vi "读取高速数据.vi"(6 "超时毫秒":i32=1000, 8 "错误输入":errorcluster caption="错误输入（无错误）", 10 "数据个数":i32, 11 "设备句柄入":i32) -> (0 "错误输出":errorcluster, 1 "返回数据个数":i32, 2 "原码值":u16[](array[numeric]), 3 "设备句柄":i32=1)   [LabVIEW 2011]
uses:
  dll/em9636.dll
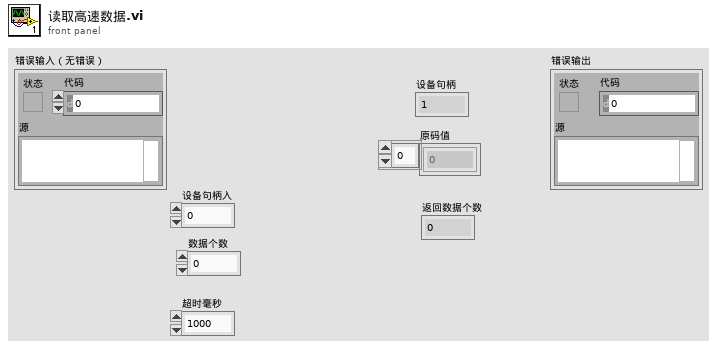
[diagram p1: front panel]
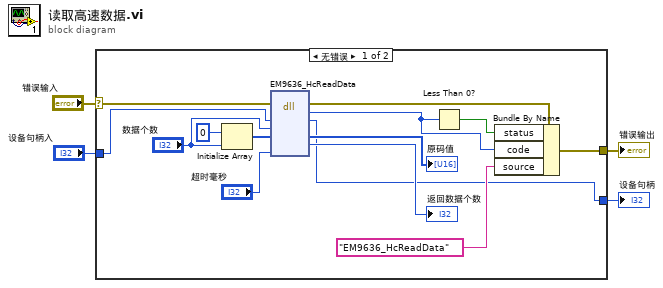
[diagram p0: block diagram]
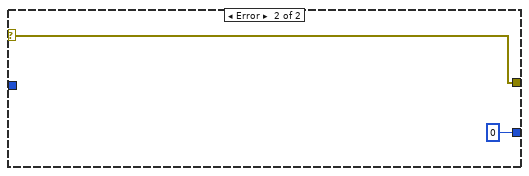
[diagram p2: hidden frame]
diagram:
  n1 = case shown="无错误" "错误输入" {
    selector: "错误输入" -> [w18 w20]
    tunnel: [w14 w20] -> w3
    tunnel: [w5 0 ("错误")] -> w2
    tunnel: "设备句柄入" -> [w12 _]
    frame No Error {
      n2 = Initialize Array(u16 0 ("元素"), "数据个数") -> (w7:u16[])
      n3 = dll-call lib="PTH1abs Eèµ éç LABVIEWæºVI(v2.0)EM9636BD)EM9636BDè°ç¨APIå½æ°æ¹æ³éè®¯ä¾ç¨EM9636labview8.5-1511048.5dll\nem9636.dll" fn="EM9636_HcReadData"(error in=w18, "设备句柄"=w12, "数据个数"="数据个数", "原码值"=w7, "超时毫秒"="超时毫秒") -> (error out=w16:errorcluster, "错误"=w13:i32, "设备句柄"=w5:i32, "原码值"=→"原码值":u16[], "返回数据个数"=→"返回数据个数":i32)  [unwired: 5 in, 1 out]
      n4 = Less Than 0?(x=w13) -> (x < 0?=w15:bool)
      n5 = Bundle By Name(cluster=w16, "status"=w15, "code"=w13, "source"="EM9636_HcReadData") -> (w14:errorcluster)
    }
    frame Error {
    }
  }
  "错误输出" <- w3
  "设备句柄" <- w2
